vi "Calc_mx+b.vi"(10 "line":cluster{"slope":dbl, "b":dbl, "theta":dbl}, 11 "point":cluster{"x":dbl, "y":dbl}) -> (3 "point on line":cluster{"x":dbl, dbl})   [LabVIEW 2022 SP3]
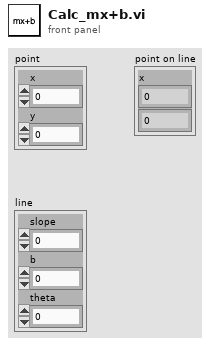
[diagram p1: front panel]
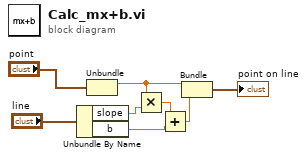
[diagram p0: block diagram]
diagram:
  n1 = Unbundle By Name("line") -> ("slope"=w2:dbl, "b"=w4:dbl)
  n2 = Unbundle("point") -> ("x"=w6:dbl)  [unwired: 1 out]
  n3 = Multiply(x=w6, y=w2) -> (x*y=w5:dbl)
  n4 = Add(x=w5, y=w4) -> (x+y=w7:dbl)
  n5 = Bundle("x"=w6, w7) -> (→"point on line":cluster{"x":dbl, dbl})  [unwired: 1 in]
